vi "Process Job.vi"(8 "error in (no error)":errorcluster, 10 "Task":refnum<class>, 11 "Stub Job Processor In":refnum<class "Stub Job Handler.lvclass">) -> (0 "error out":errorcluster, 3 "Stub Job Processor Out":refnum<class "Stub Job Handler.lvclass">)   [LabVIEW 2020, in "Stub Job Handler.lvclass"]
uses:
  Stub Job Handler.lvclass
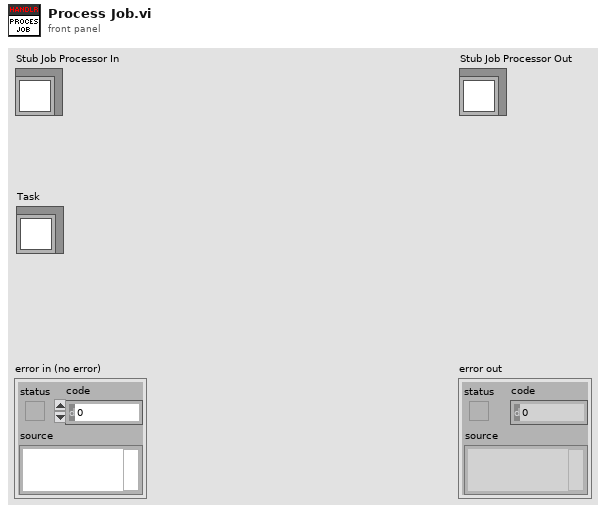
[diagram p1: front panel]
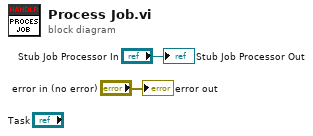
[diagram p0: block diagram]
diagram:
  "error out" <- "error in (no error)"
  "Stub Job Processor Out" <- "Stub Job Processor In"
